vi "Staib EG.vi"(0 "QUIT":refnum<vi>, 1 "Scan in Progress":refnum<vi>, 2 "Set EG":refnum<vi>, 3 "Energy (eV)":refnum<vi>, 4 "Extraction (V)":refnum<vi>, 5 "Filament (V)":refnum<vi>, 6 "EG Computer Control":refnum<vi>, 7 "X1 Alignment (V)":refnum<vi>, 8 "Error":refnum<vi>, 9 "X2 Alignment (V)":refnum<vi>, 11 "Y1 Alignment (V)":refnum<vi>, 13 "Y2 Alignment (V)":refnum<vi>, 14 "Grid (V)":refnum<vi>, 15 "Focus 1 (V)":refnum<vi>, 16 "Focus 2 (V)":refnum<vi>) -> ()   [LabVIEW 2010]
uses:
  <vilib>/DAQmx/write.llb/DAQmx Write (Analog DBL 1Chan 1Samp).vi
  <vilib>/DAQmx/write.llb/DAQmx Write (Digital Bool 1Line 1Point).vi
  <vilib>/daqmx/miscellaneous.llb/DAQmx Fill In Error Info.vi
panel:
  in  "Staib Electron Gun":enum32{"Controls", "Settings"}(tab)
  in  "Lock Focus Knobs":bool
  out "Computer\nControl Enabled?":bool
  in  "Computer\nControl":bool
  in  "Y2 Alignment (V)":dbl(knob) min=-10.0 max=10.0 step=0.001 scale=-10.0..10.0 scale format="%#_3g"
  in  "Y1 Alignment (V)":dbl(knob) min=-10.0 max=10.0 step=0.001 scale=-10.0..10.0 scale format="%#_3g"
  in  "X2 Alignment (V)":dbl(knob) min=-10.0 max=10.0 step=0.001 scale=-10.0..10.0 scale format="%#_3g"
  in  "X1 Alignment (V)":dbl(knob) min=-10.0 max=10.0 step=0.001 scale=-10.0..10.0 scale format="%#_3g"
  in  "Filament (V)":dbl(knob) min=0.0 max=10.0 step=0.001 scale=0.0..5.0 scale format="%#_3g"
  in  "Focus 2 (V)":dbl(knob) min=-0.0 max=0.0 step=0.001 scale=0.0..0.001 scale format="%#_3g"
  in  "Focus 1 (V)":dbl(knob) min=-0.0 max=0.0 step=0.001 scale=0.0..0.001 scale format="%#_3g"
  in  "Extraction (V)":dbl(knob) min=0.0 max=100.0 step=0.001 scale=0.0..100.0 scale format="%#_3g"
  in  "Energy (eV)":dbl(knob) min=0.0 max=100.0 step=0.001 scale=0.0..100.0 scale format="%#_3g"
  in  "Grid (V)":dbl(knob) min=-15.0 max=15.0 step=0.001 scale=-15.0..15.0 scale format="%#_3g"
  out "Feedback Extraction":dbl caption="Ext"
  out "Feedback Filament":dbl caption="Fil"
  out "Feedback Energy":dbl caption="En"
  out "Feedback Grid":dbl caption="G"
  out "Feedback Focus 1":dbl caption="F 1"
  out "Feedback Focus 2":dbl caption="F 2"
  out "Feedback X1 Alignment":dbl caption="X1"
  out "Feedback X2 Alignment":dbl caption="X2"
  out "Feedback Y1 Alignment":dbl caption="Y1"
  out "Feedback Y2 Alignment":dbl caption="Y2"
  out "Focus Max (V)":dbl min=0.0 max=100.0 step=0.001
  out "Focus Min (V)":dbl
  out "Focus Disable":i32
  in  "Minimum Upper Limit of Focus' Scale (V)":dbl=0.001 min=1e-05 max=100.0 step=0.001
  # "Note that there is no feedback from the electron gun's hardware.  Check the controller's LEDs if unsure."
  # "On"
  # "Off"
  # "Software Feedback"
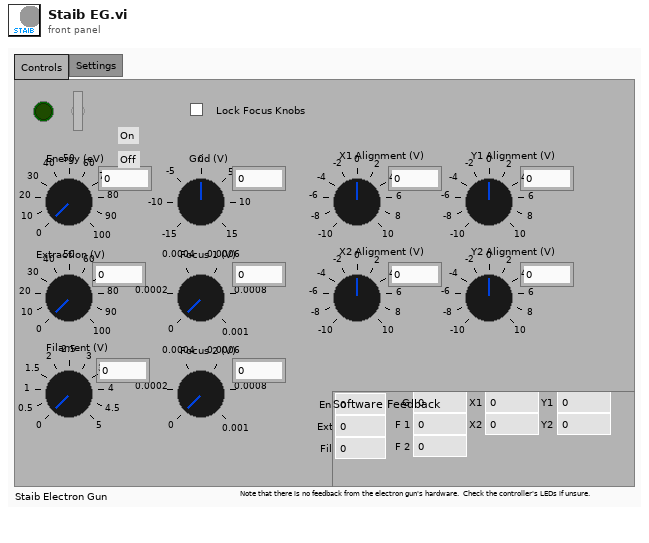
[diagram p1: front panel]
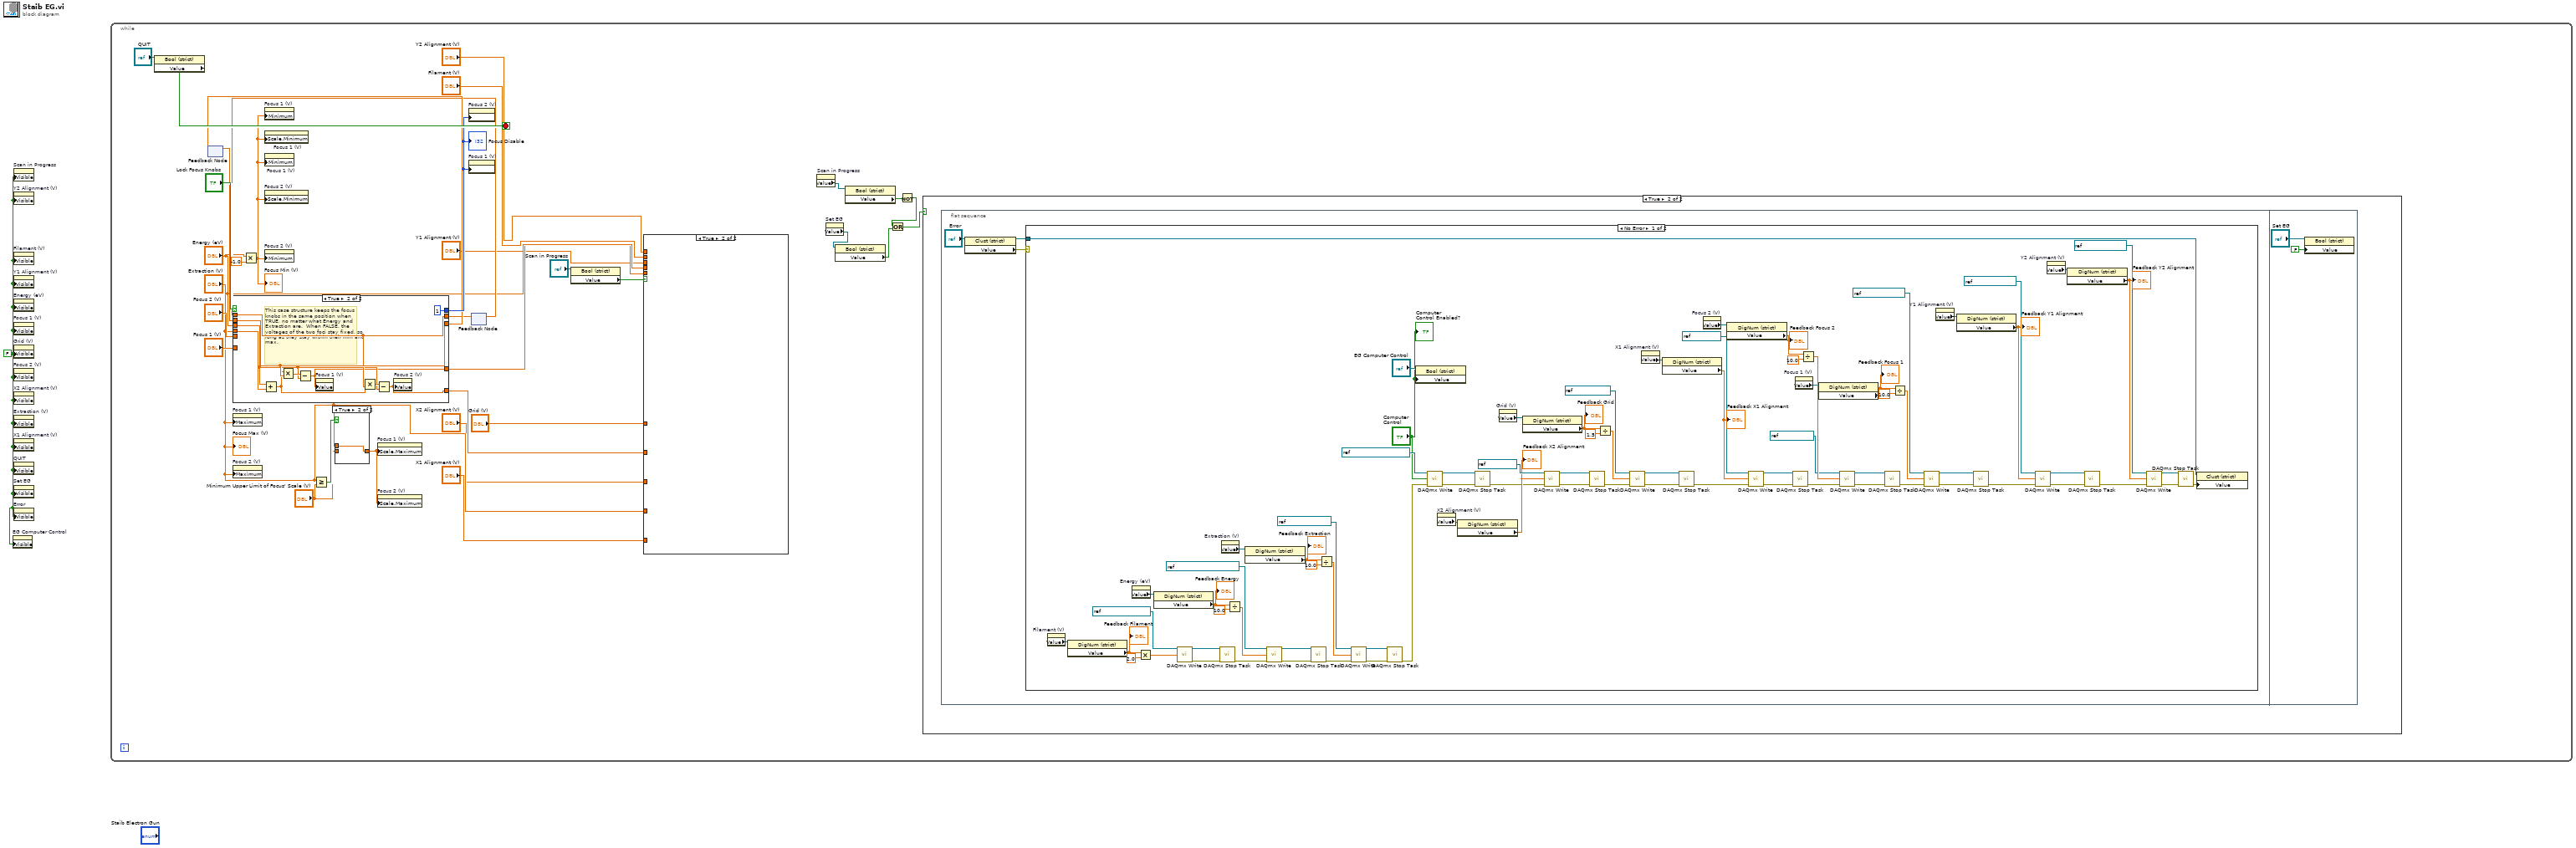
[diagram p0: block diagram]
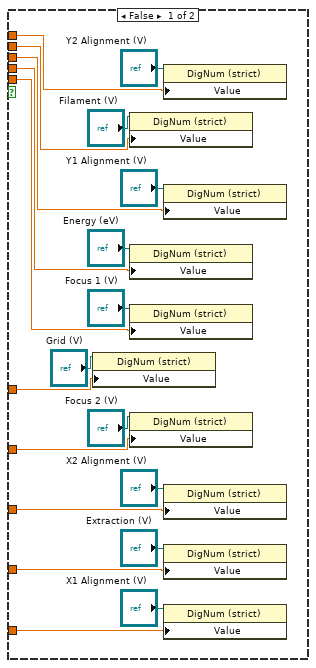
[diagram p4: hidden frame]
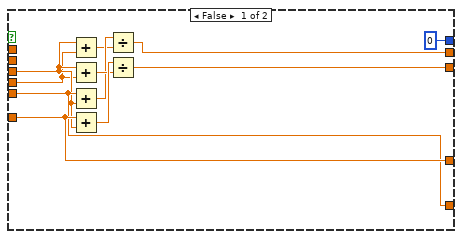
[diagram p6: hidden frame]
diagram:
  w1 = FALSE ("Visible")
  n1 = property on="EG Computer Control" class="LVObjRef (strict)"("Visible"=w1) -> ()  [unwired: 2 in, 2 out]
  n2 = property on="Scan in Progress" class="LVObjRef (strict)"("Visible"=w1) -> ()  [unwired: 2 in, 2 out]
  n3 = property on="Y2 Alignment (V)" class="LVObjRef (strict)"("Visible"=w1) -> ()  [unwired: 2 in, 2 out]
  n4 = property on="Filament (V)" class="LVObjRef (strict)"("Visible"=w1) -> ()  [unwired: 2 in, 2 out]
  n5 = property on="Y1 Alignment (V)" class="LVObjRef (strict)"("Visible"=w1) -> ()  [unwired: 2 in, 2 out]
  n6 = property on="Energy (eV)" class="LVObjRef (strict)"("Visible"=w1) -> ()  [unwired: 2 in, 2 out]
  n7 = property on="Focus 1 (V)" class="LVObjRef (strict)"("Visible"=w1) -> ()  [unwired: 2 in, 2 out]
  n8 = property on="Grid (V)" class="LVObjRef (strict)"("Visible"=w1) -> ()  [unwired: 2 in, 2 out]
  n9 = property on="Focus 2 (V)" class="LVObjRef (strict)"("Visible"=w1) -> ()  [unwired: 2 in, 2 out]
  n10 = property on="X2 Alignment (V)" class="LVObjRef (strict)"("Visible"=w1) -> ()  [unwired: 2 in, 2 out]
  n11 = property on="Extraction (V)" class="LVObjRef (strict)"("Visible"=w1) -> ()  [unwired: 2 in, 2 out]
  n12 = property on="X1 Alignment (V)" class="LVObjRef (strict)"("Visible"=w1) -> ()  [unwired: 2 in, 2 out]
  n13 = property on="QUIT" class="LVObjRef (strict)"("Visible"=w1) -> ()  [unwired: 2 in, 2 out]
  n14 = property on="Set EG" class="LVObjRef (strict)"("Visible"=w1) -> ()  [unwired: 2 in, 2 out]
  n15 = property on="Error" class="LVObjRef (strict)"("Visible"=w1) -> ()  [unwired: 2 in, 2 out]
  n16 = while {
    stop <- w33 stop-if-true
    n17 = property class="Bool (strict)"(reference="QUIT") -> ("Value"=w33:bool)  [unwired: 1 in, 2 out]
    n18 = feedback #1() -> (w26:dbl)  [unwired: 1 in]
    n19 = property on="Focus 1 (V)" class="Knob (strict)"("Maximum"="Extraction (V)") -> ()  [unwired: 2 in, 2 out]
    n20 = property on="Focus 2 (V)" class="Knob (strict)"("Maximum"="Extraction (V)") -> ()  [unwired: 2 in, 2 out]
    n21 = Multiply(x="Energy (eV)", y=-1.0) -> (x*y=w21:dbl)
    "Focus Min (V)" <- w21
    n22 = property on="Focus 1 (V)" class="Knob (strict)"("Minimum"=w21) -> ()  [unwired: 2 in, 2 out]
    n23 = property on="Focus 1 (V)" class="Knob (strict)"("Scale.Minimum"=w21) -> ()  [unwired: 2 in, 2 out]
    n24 = property on="Focus 1 (V)" class="Knob (strict)"("Minimum"=w21) -> ()  [unwired: 2 in, 2 out]
    n25 = property on="Focus 2 (V)" class="Knob (strict)"("Scale.Minimum"=w21) -> ()  [unwired: 2 in, 2 out]
    n26 = property on="Focus 2 (V)" class="Knob (strict)"("Minimum"=w21) -> ()  [unwired: 2 in, 2 out]
    n27 = Greater Or Equal?(x="Extraction (V)", y="Minimum Upper Limit of Focus' Scale (V)") -> (x >= y?=w23:bool)
    n28 = case shown="True" w23 {
      tunnel: "Extraction (V)" -> [_ w140]
      tunnel: [w139 w140] -> w22
      tunnel: "Minimum Upper Limit of Focus' Scale (V)" -> [w139 _]
      frame False {
      }
      frame True {
      }
    }
    n29 = property on="Focus 1 (V)" class="Knob (strict)"("Scale.Maximum"=w22) -> ()  [unwired: 2 in, 2 out]
    n30 = property on="Focus 2 (V)" class="Knob (strict)"("Scale.Maximum"=w22) -> ()  [unwired: 2 in, 2 out]
    n31 = feedback #2() -> (w24:dbl)  [unwired: 1 in]
    n32 = case shown="True" "Lock Focus Knobs" {
      tunnel: "Focus 2 (V)" -> [w144 _]
      tunnel: [w144 w152] -> w14
      tunnel: "Focus 1 (V)" -> [w150 _]
      tunnel: [w150 w153] -> w15
      tunnel: [0 1] -> w30
      tunnel: "Energy (eV)" -> [w143 w154]
      tunnel: "Extraction (V)" -> [w142 w160]
      tunnel: [w147 w158] -> w27
      tunnel: [w141 w156] -> w25
      tunnel: w26 -> [_ w158]
      tunnel: w24 -> [_ w156]
      frame False {
        n33 = Add(x=w143, y=w142) -> (x+y=w145:dbl)
        n34 = Add(x=w143, y=w142) -> (x+y=w148:dbl)
        n35 = Add(x=w144, y=w143) -> (x+y=w146:dbl)
        n36 = Add(x=w150, y=w143) -> (x+y=w149:dbl)
        n37 = Divide(x=w146, y=w145) -> (x/y=w141:dbl)
        n38 = Divide(x=w149, y=w148) -> (x/y=w147:dbl)
      }
      frame True {
        # "This case structure keeps the focus knobs in the same position when TRUE, no matter what Energy and Extraction are.  When FALSE, the voltages of the two foci stay fixed, so long as they stay within their min and max."
        n39 = Add(x=w154, y=w160) -> (x+y=w157:dbl)
        n40 = Multiply(x=w157, y=w158) -> (x*y=w159:dbl)
        n41 = Subtract(x=w159, y=w154) -> (x-y=w153:dbl)
        n42 = property on="Focus 1 (V)" class="Knob (strict)"("Value"=w153) -> ()  [unwired: 2 in, 2 out]
        n43 = Multiply(x=w157, y=w156) -> (x*y=w155:dbl)
        n44 = Subtract(x=w155, y=w154) -> (x-y=w152:dbl)
        n45 = property on="Focus 2 (V)" class="Knob (strict)"("Value"=w152) -> ()  [unwired: 2 in, 2 out]
      }
    }
    "Focus Disable" <- w30
    n46 = feedback-in #1(w27) -> ()
    n47 = property on="Focus 2 (V)" class="Knob (strict)"("DisabledEnum"=w30) -> ()  [unwired: 2 in, 2 out]
    n48 = property on="Focus 1 (V)" class="Knob (strict)"("DisabledEnum"=w30) -> ()  [unwired: 2 in, 2 out]
    n49 = feedback-in #2(w25) -> ()
    n50 = property class="Bool (strict)"(reference="Scan in Progress") -> ("Value"=w8:bool)  [unwired: 1 in, 2 out]
    n51 = case shown="True" w8 {
      tunnel: "Energy (eV)" -> [w138 _]
      tunnel: "Extraction (V)" -> [w137 _]
      tunnel: "Filament (V)" -> [w136 _]
      tunnel: "Grid (V)" -> [w135 _]
      tunnel: w15 -> [w134 _]
      tunnel: w14 -> [w133 _]
      tunnel: "X1 Alignment (V)" -> [w132 _]
      tunnel: "X2 Alignment (V)" -> [w131 _]
      tunnel: "Y1 Alignment (V)" -> [w130 _]
      tunnel: "Y2 Alignment (V)" -> [w129 _]
      frame False {
        n52 = property class="DigNum (strict)"(reference="Grid (V)", "Value"=w135) -> ()  [unwired: 1 in, 2 out]
        n53 = property class="DigNum (strict)"(reference="Filament (V)", "Value"=w136) -> ()  [unwired: 1 in, 2 out]
        n54 = property class="DigNum (strict)"(reference="Energy (eV)", "Value"=w138) -> ()  [unwired: 1 in, 2 out]
        n55 = property class="DigNum (strict)"(reference="Focus 1 (V)", "Value"=w134) -> ()  [unwired: 1 in, 2 out]
        n56 = property class="DigNum (strict)"(reference="Focus 2 (V)", "Value"=w133) -> ()  [unwired: 1 in, 2 out]
        n57 = property class="DigNum (strict)"(reference="Y2 Alignment (V)", "Value"=w129) -> ()  [unwired: 1 in, 2 out]
        n58 = property class="DigNum (strict)"(reference="Y1 Alignment (V)", "Value"=w130) -> ()  [unwired: 1 in, 2 out]
        n59 = property class="DigNum (strict)"(reference="X2 Alignment (V)", "Value"=w131) -> ()  [unwired: 1 in, 2 out]
        n60 = property class="DigNum (strict)"(reference="Extraction (V)", "Value"=w137) -> ()  [unwired: 1 in, 2 out]
        n61 = property class="DigNum (strict)"(reference="X1 Alignment (V)", "Value"=w132) -> ()  [unwired: 1 in, 2 out]
      }
      frame True {
      }
    }
    n62 = property on="Scan in Progress" class="LVObjRef (strict)"() -> ("Value"=w7:refnum<vi>)  [unwired: 2 in, 2 out]
    n63 = property on="Set EG" class="LVObjRef (strict)"() -> ("Value"=w5:refnum<vi>)  [unwired: 2 in, 2 out]
    n64 = property class="Bool (strict)"(reference=w5) -> ("Value"=w4:bool)  [unwired: 1 in, 2 out]
    n65 = property class="Bool (strict)"(reference=w7) -> ("Value"=w6:bool)  [unwired: 1 in, 2 out]
    n66 = Not(x=w6) -> (.not. x?=w2:bool)
    n67 = Or(x=w2, y=w4) -> (x .or. y?=w3:bool)
    n68 = case shown="True" w3 {
      frame False {
      }
      frame True {
        n69 = flat-sequence {
          frame #0 {
            n70 = property class="Clust (strict)"(reference="Error") -> (reference out=w36:refnum<vi>, "Value"=w35:errorcluster)  [unwired: 1 in, 1 out]
            n71 = case shown="No Error" w35 {
              tunnel: w36 -> [w60 _]
              frame No Error {
                n72 = property on="Filament (V)" class="LVObjRef (strict)"() -> ("Value"=w93:refnum<vi>)  [unwired: 2 in, 2 out]
                n73 = property class="DigNum (strict)"(reference=w93) -> ("Value"=w83:dbl)  [unwired: 1 in, 2 out]
                "Feedback Filament" <- w83
                n74 = property on="Energy (eV)" class="LVObjRef (strict)"() -> ("Value"=w92:refnum<vi>)  [unwired: 2 in, 2 out]
                n75 = Multiply(x=w83, y=2.0) -> (x*y=w108:dbl)
                n76 = property class="DigNum (strict)"(reference=w92) -> ("Value"=w82:dbl)  [unwired: 1 in, 2 out]
                "Feedback Energy" <- w82
                n77 = call-poly <vilib>:"DAQmx Write.vi"("task/channels in"=refnum<k21> "Filament out", "data"=w108) -> ("task out"=w70:refnum<k21>, "error out"=w59:errorcluster)  [unwired: 11 in, 1 out]
                n78 = call <vilib>:"DAQmx Stop Task.vi"("task/channels in"=w70, "error in"=w59) -> ("error out"=w58:errorcluster)  [unwired: 12 in, 1 out]
                n79 = property on="Extraction (V)" class="LVObjRef (strict)"() -> ("Value"=w91:refnum<vi>)  [unwired: 2 in, 2 out]
                n80 = Divide(x=w82, y=10.0) -> (x/y=w111:dbl)
                n81 = property class="DigNum (strict)"(reference=w91) -> ("Value"=w81:dbl)  [unwired: 1 in, 2 out]
                "Feedback Extraction" <- w81
                n82 = call-poly <vilib>:"DAQmx Write.vi"("task/channels in"=refnum<k21> "Electron Energy Out", "data"=w111, "error in"=w58) -> ("task out"=w69:refnum<k21>, "error out"=w57:errorcluster)  [unwired: 10 in, 1 out]
                n83 = call <vilib>:"DAQmx Stop Task.vi"("task/channels in"=w69, "error in"=w57) -> ("error out"=w56:errorcluster)  [unwired: 12 in, 1 out]
                n84 = Divide(x=w81, y=10.0) -> (x/y=w106:dbl)
                n85 = call-poly <vilib>:"DAQmx Write.vi"("task/channels in"=refnum<k21> "Extraction out", "data"=w106, "error in"=w56) -> ("task out"=w68:refnum<k21>, "error out"=w55:errorcluster)  [unwired: 10 in, 1 out]
                n86 = call <vilib>:"DAQmx Stop Task.vi"("task/channels in"=w68, "error in"=w55) -> ("error out"=w54:errorcluster)  [unwired: 12 in, 1 out]
                n87 = property class="Bool (strict)"(reference="EG Computer Control", "Value"="Computer\nControl") -> ()  [unwired: 1 in, 2 out]
                n88 = call-poly <vilib>:"DAQmx Write.vi"("task/channels in"=refnum<k21> "ElectronCPUControl", "data"="Computer\nControl", "error in"=w54) -> ("task out"=w67:refnum<k21>, "error out"=w53:errorcluster)  [unwired: 10 in, 1 out]
                n89 = property on="X2 Alignment (V)" class="LVObjRef (strict)"() -> ("Value"=w90:refnum<vi>)  [unwired: 2 in, 2 out]
                n90 = property class="DigNum (strict)"(reference=w90) -> ("Value"=w80:dbl)  [unwired: 1 in, 2 out]
                "Feedback X2 Alignment" <- w80
                n91 = call <vilib>:"DAQmx Stop Task.vi"("task/channels in"=w67, "error in"=w53) -> ("error out"=w52:errorcluster)  [unwired: 12 in, 1 out]
                n92 = property on="Grid (V)" class="LVObjRef (strict)"() -> ("Value"=w89:refnum<vi>)  [unwired: 2 in, 2 out]
                n93 = property class="DigNum (strict)"(reference=w89) -> ("Value"=w79:dbl)  [unwired: 1 in, 2 out]
                "Feedback Grid" <- w79
                n94 = call-poly <vilib>:"DAQmx Write.vi"("task/channels in"=refnum<k21> "X2 out", "data"=w80, "error in"=w52) -> ("task out"=w66:refnum<k21>, "error out"=w51:errorcluster)  [unwired: 10 in, 1 out]
                n95 = call <vilib>:"DAQmx Stop Task.vi"("task/channels in"=w66, "error in"=w51) -> ("error out"=w50:errorcluster)  [unwired: 12 in, 1 out]
                n96 = Divide(x=w79, y=1.5) -> (x/y=w104:dbl)
                n97 = call-poly <vilib>:"DAQmx Write.vi"("task/channels in"=refnum<k21> "Grid Out", "data"=w104, "error in"=w50) -> ("task out"=w65:refnum<k21>, "error out"=w49:errorcluster)  [unwired: 10 in, 1 out]
                n98 = property on="X1 Alignment (V)" class="LVObjRef (strict)"() -> ("Value"=w88:refnum<vi>)  [unwired: 2 in, 2 out]
                n99 = property class="DigNum (strict)"(reference=w88) -> ("Value"=w78:dbl)  [unwired: 1 in, 2 out]
                "Feedback X1 Alignment" <- w78
                n100 = call <vilib>:"DAQmx Stop Task.vi"("task/channels in"=w65, "error in"=w49) -> ("error out"=w48:errorcluster)  [unwired: 12 in, 1 out]
                n101 = property on="Focus 2 (V)" class="LVObjRef (strict)"() -> ("Value"=w87:refnum<vi>)  [unwired: 2 in, 2 out]
                n102 = property class="DigNum (strict)"(reference=w87) -> ("Value"=w77:dbl)  [unwired: 1 in, 2 out]
                "Feedback Focus 2" <- w77
                n103 = call-poly <vilib>:"DAQmx Write.vi"("task/channels in"=refnum<k21> "X1 out", "data"=w78, "error in"=w48) -> ("task out"=w64:refnum<k21>, "error out"=w47:errorcluster)  [unwired: 10 in, 1 out]
                n104 = call <vilib>:"DAQmx Stop Task.vi"("task/channels in"=w64, "error in"=w47) -> ("error out"=w46:errorcluster)  [unwired: 12 in, 1 out]
                n105 = property on="Focus 1 (V)" class="LVObjRef (strict)"() -> ("Value"=w86:refnum<vi>)  [unwired: 2 in, 2 out]
                n106 = Divide(x=w77, y=10.0) -> (x/y=w115:dbl)
                n107 = property class="DigNum (strict)"(reference=w86) -> ("Value"=w76:dbl)  [unwired: 1 in, 2 out]
                "Feedback Focus 1" <- w76
                n108 = call-poly <vilib>:"DAQmx Write.vi"("task/channels in"=refnum<k21> "Focus 2 out", "data"=w115, "error in"=w46) -> ("task out"=w63:refnum<k21>, "error out"=w45:errorcluster)  [unwired: 10 in, 1 out]
                n109 = call <vilib>:"DAQmx Stop Task.vi"("task/channels in"=w63, "error in"=w45) -> ("error out"=w44:errorcluster)  [unwired: 12 in, 1 out]
                n110 = Divide(x=w76, y=10.0) -> (x/y=w116:dbl)
                n111 = call-poly <vilib>:"DAQmx Write.vi"("task/channels in"=refnum<k21> "Focus 1 out", "data"=w116, "error in"=w44) -> ("task out"=w62:refnum<k21>, "error out"=w43:errorcluster)  [unwired: 10 in, 1 out]
                n112 = property on="Y1 Alignment (V)" class="LVObjRef (strict)"() -> ("Value"=w85:refnum<vi>)  [unwired: 2 in, 2 out]
                n113 = property class="DigNum (strict)"(reference=w85) -> ("Value"=w75:dbl)  [unwired: 1 in, 2 out]
                "Feedback Y1 Alignment" <- w75
                n114 = call <vilib>:"DAQmx Stop Task.vi"("task/channels in"=w62, "error in"=w43) -> ("error out"=w42:errorcluster)  [unwired: 12 in, 1 out]
                n115 = call-poly <vilib>:"DAQmx Write.vi"("task/channels in"=refnum<k21> "Y1 out", "data"=w75, "error in"=w42) -> ("task out"=w71:refnum<k21>, "error out"=w41:errorcluster)  [unwired: 10 in, 1 out]
                n116 = property on="Y2 Alignment (V)" class="LVObjRef (strict)"() -> ("Value"=w84:refnum<vi>)  [unwired: 2 in, 2 out]
                n117 = property class="DigNum (strict)"(reference=w84) -> ("Value"=w74:dbl)  [unwired: 1 in, 2 out]
                "Feedback Y2 Alignment" <- w74
                n118 = call <vilib>:"DAQmx Stop Task.vi"("task/channels in"=w71, "error in"=w41) -> ("error out"=w40:errorcluster)  [unwired: 12 in, 1 out]
                n119 = call-poly <vilib>:"DAQmx Write.vi"("task/channels in"=refnum<k21> "Y2 out", "data"=w74, "error in"=w40) -> ("task out"=w61:refnum<k21>, "error out"=w39:errorcluster)  [unwired: 10 in, 1 out]
                n120 = call <vilib>:"DAQmx Stop Task.vi"("task/channels in"=w61, "error in"=w39) -> ("error out"=w38:errorcluster)  [unwired: 12 in, 1 out]
                n121 = property class="Clust (strict)"(reference=w60, "Value"=w38) -> ()  [unwired: 1 in, 2 out]
                "Computer\nControl Enabled?" <- "Computer\nControl"
              }
              frame Error {
              }
            }
          }
          frame #1 {
            n122 = property class="Bool (strict)"(reference="Set EG", "Value"=FALSE) -> ()  [unwired: 1 in, 2 out]
          }
        }
      }
    }
    "Focus Max (V)" <- "Extraction (V)"
  }
